vi "Polymorphic Add.vi"() -> ()   [LabVIEW 2012]
panel:
  out "Array":i32[](array[numeric])
  out "Array":i32[](array[numeric])
  out "Scalar":i32
  out "Array":i32[](array[numeric])
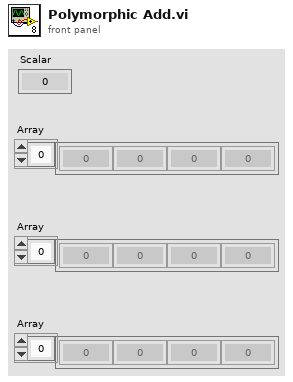
[diagram p1: front panel]
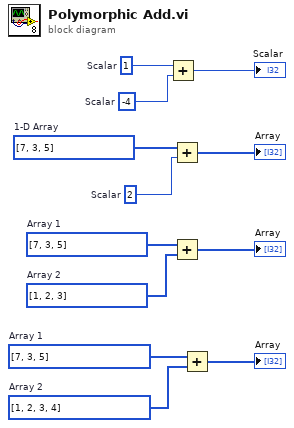
[diagram p0: block diagram]
diagram:
  w2 = i32[] [1, 2, 3, 4]  # Array 2
  w3 = i32[] [7, 3, 5]  # Array 1
  w7 = i32[] [1, 2, 3]  # Array 2
  w6 = i32[] [7, 3, 5]  # Array 1
  w12 = 1  # Scalar
  w9 = i32[] [7, 3, 5]  # 1-D Array
  w8 = 2  # Scalar
  w11 = -4  # Scalar
  n1 = Add(x=w12, y=w11) -> (x+y=→"Scalar":i32)
  n2 = Add(x=w9, y=w8) -> (x+y=→"Array":i32[])
  n3 = Add(x=w6, y=w7) -> (x+y=→"Array":i32[])
  n4 = Add(x=w3, y=w2) -> (x+y=→"Array":i32[])
